vi "Read Database.vi"(8 "error in (no error)":errorcluster, 11 "Postgres Connector in":refnum<class "Postgres Connector.lvclass">) -> (0 "error out":errorcluster, 2 "Database":string, 3 "Postgres Connector out":refnum<class "Postgres Connector.lvclass">)   [LabVIEW 2020, in "Postgres Connector.lvclass"]
uses:
  Postgres Connector.lvclass
  Postgres Connector.lvclass/Postgres Connector.ctl
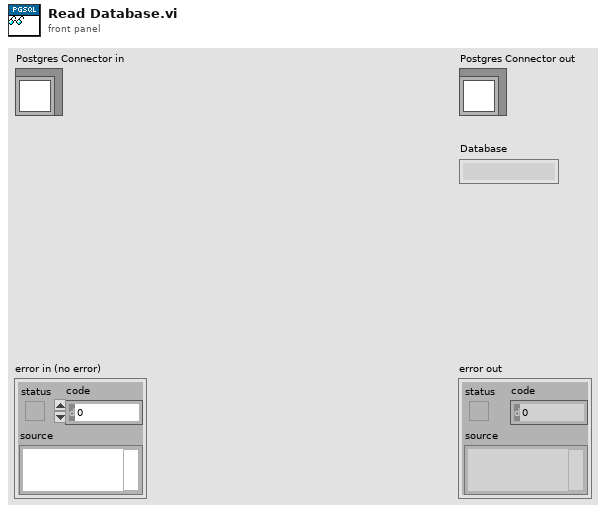
[diagram p1: front panel]
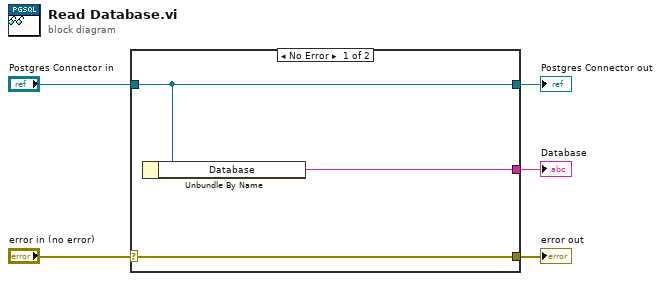
[diagram p0: block diagram]
diagram:
  n1 = case shown="No Error" "error in (no error)" {
    selector: "error in (no error)" -> [w8 w9]
    tunnel: [w8 w9] -> w4
    tunnel: [w7 w10] -> w2
    tunnel: "Postgres Connector in" -> [w7 w10]
    tunnel: [w6 _] -> w1
    frame No Error {
      n2 = Unbundle By Name(w7) -> ("Database"=w6:string)
    }
    frame Error {
    }
  }
  "error out" <- w4
  "Postgres Connector out" <- w2
  "Database" <- w1
